vi "Run Dual Mode Thermometer XControl.vi"() -> ()   [LabVIEW 2023]
doc: "This VI demonstrates the functionality of the Dual Mode Thermometer XControl. \n\nUsing different combinations of the mode on the DMTC and the DMTI will demonstrate the Dual Mode Thermometer XControl's functionality. The Fahrenheit Mode? boolean is indicating whether the DMTI is in Fahrenheit mode by using a custom Property created for the DMT XControl. The Converter converts Celsius to Fahrenheit using a Convert C to F method created for the DMT XControl. Refer to the Project Explorer and the XControl Help for more information on XControls."
uses:
  Simple Dual Mode Thermometer XControl.xctl
panel:
  out "Degrees Fahrenheit":dbl
  in  "Degrees Celsius":dbl
  out "Fahrenheit?":bool
  out "Dual Mode Thermometer Indicator (DMTI)":dbl(xcontrol)=28.09917355371901
  in  "Dual Mode Thermometer Control (DMTC)":dbl(xcontrol)=28.09917355371901
  in  "Stop":bool
  # "Overview: This VI demonstrates the functionality of the Dual Mode Thermometer XControl.\nInstructions:\n1. Run the VI.\n2. Adjust the DMTC.\n3. Select the Fahrenheit mode of DMTC.\n4. Adjust the DMTC.\n5. Select the Fahrenheit mode of DMTI.\n6. Adjust the DMTC.\n7. Click Stop to stop the VI.\n\nNote: Close this VI before attempting to make any changes to the Dual Mode Thermometer XControl."
  # "Temperature Converter"
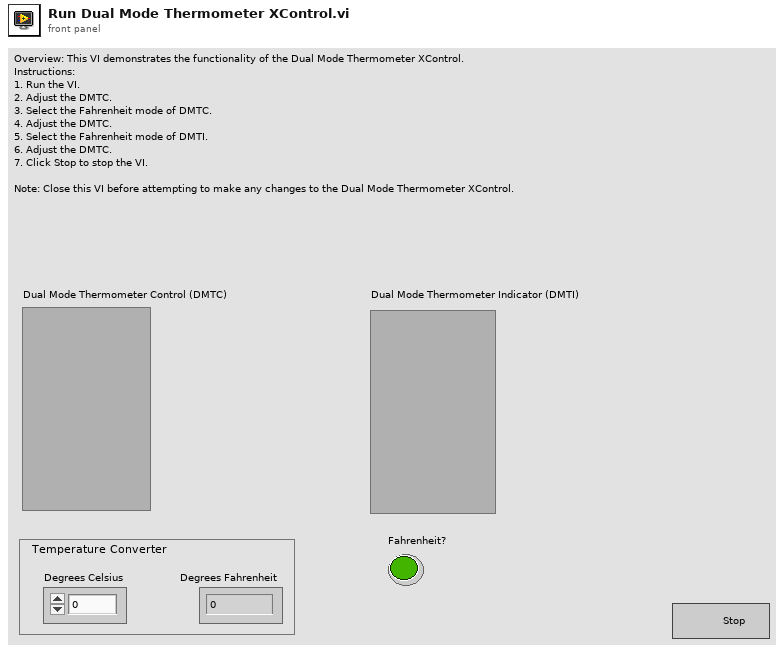
[diagram p1: front panel]
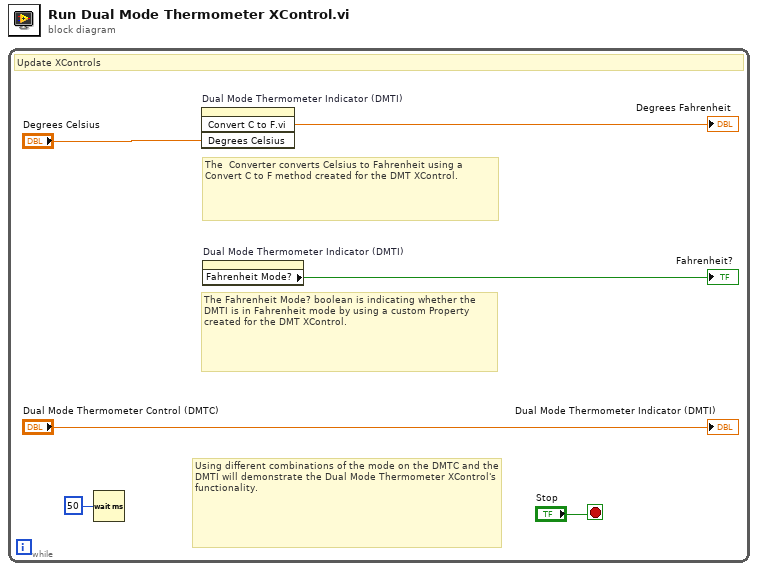
[diagram p0: block diagram]
diagram:
  n1 = while {
    stop <- "Stop" stop-if-true
    # "Using different combinations of the mode on the DMTC and the DMTI will demonstrate the Dual Mode Thermometer XControl's functionality."
    # "The  Converter converts Celsius to Fahrenheit using a Convert C to F method created for the DMT XControl."
    # "The Fahrenheit Mode? boolean is indicating whether the DMTI is in Fahrenheit mode by using a custom Property created for the DMT XControl."
    # "Update XControls"
    n2 = Wait (ms)(milliseconds to wait=u32 50) -> ()  [unwired: 1 out]
    n3 = invoke on="Dual Mode Thermometer Indicator (DMTI)" class="Simple Dual Mode Thermometer XC" method="Convert C to F.vi"("Degrees Celsius"="Degrees Celsius") -> ("Convert C to F.vi"=→"Degrees Fahrenheit":dbl)  [unwired: 3 in, 3 out]
    n4 = property on="Dual Mode Thermometer Indicator (DMTI)" class="Simple Dual Mode Thermometer XC"() -> ("Fahrenheit Mode?"=→"Fahrenheit?":bool)  [unwired: 2 in, 2 out]
    "Dual Mode Thermometer Indicator (DMTI)" <- "Dual Mode Thermometer Control (DMTC)"
  }
